vi "Surface_modularity.vi"(2 "Data in":string[][](array[string]), 3 "Channel names":string[](array[string])) -> (0 "Data out":string[][](array[string]))   [LabVIEW 2018]
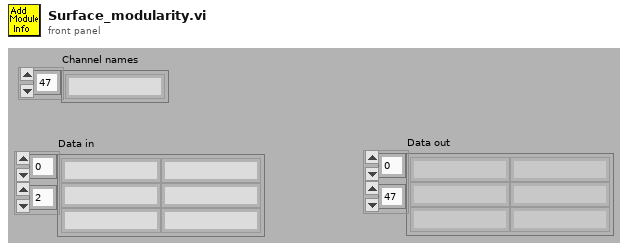
[diagram p1: front panel]
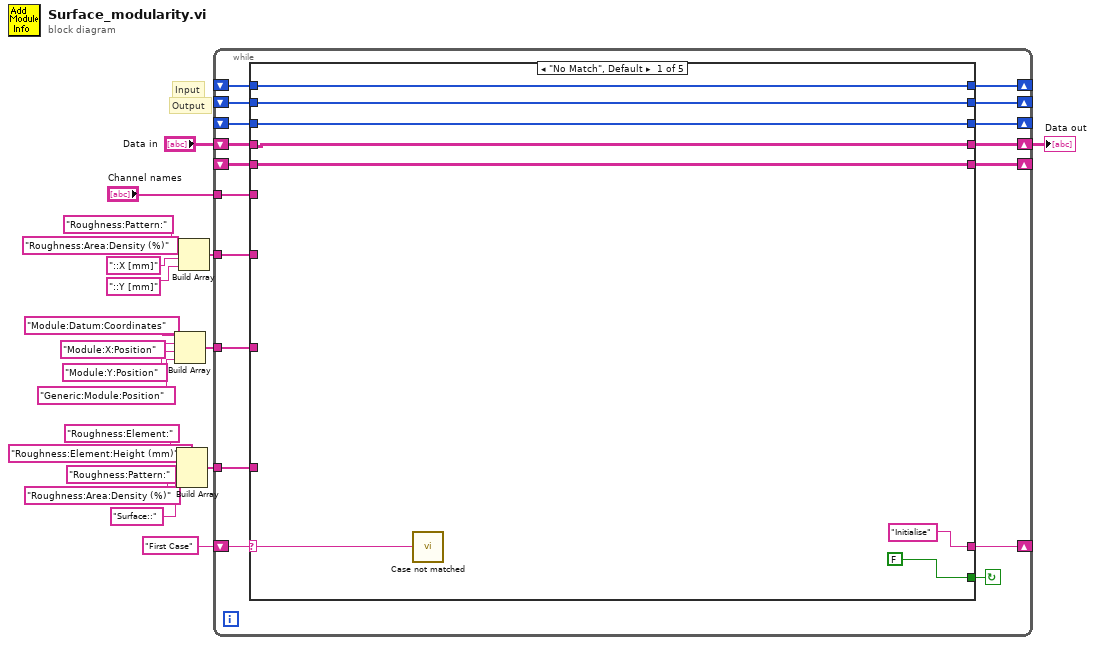
[diagram p0: block diagram]
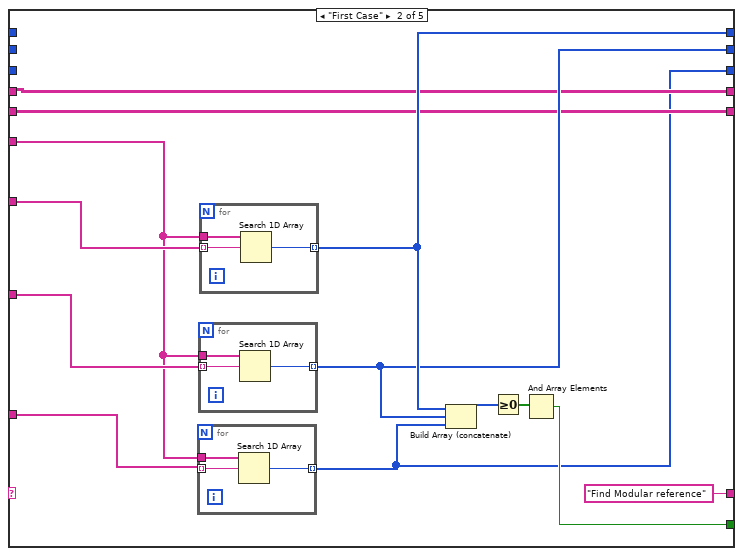
[diagram p2: hidden frame]
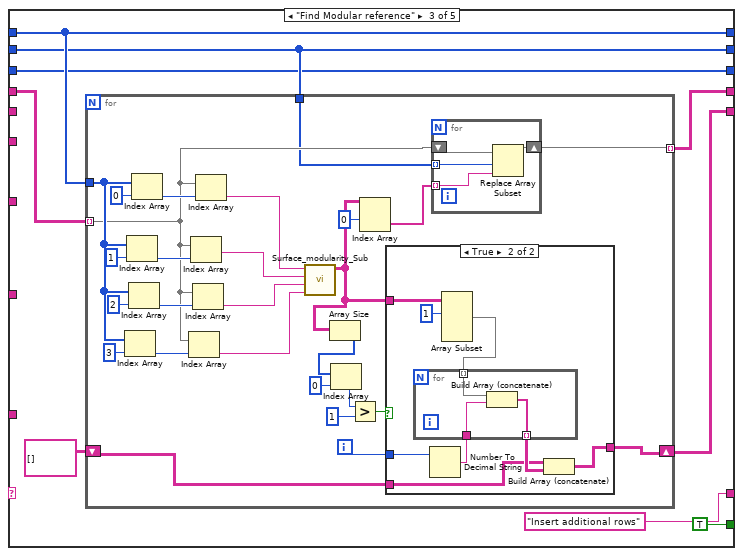
[diagram p3: hidden frame]
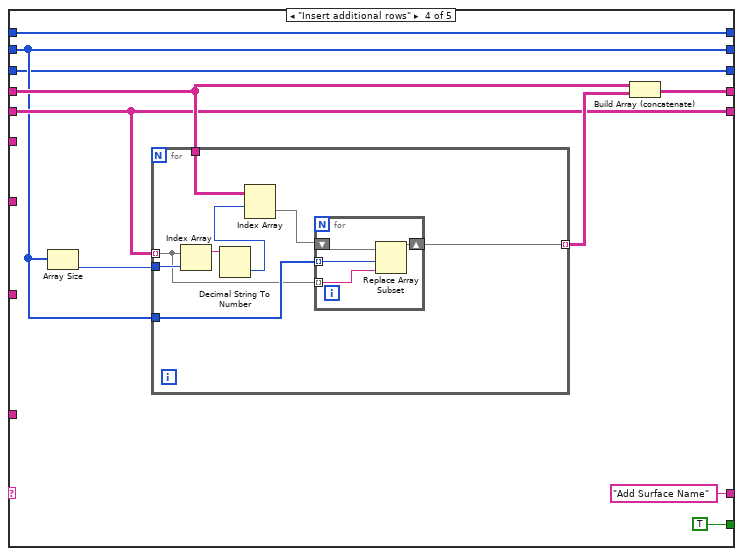
[diagram p5: hidden frame]
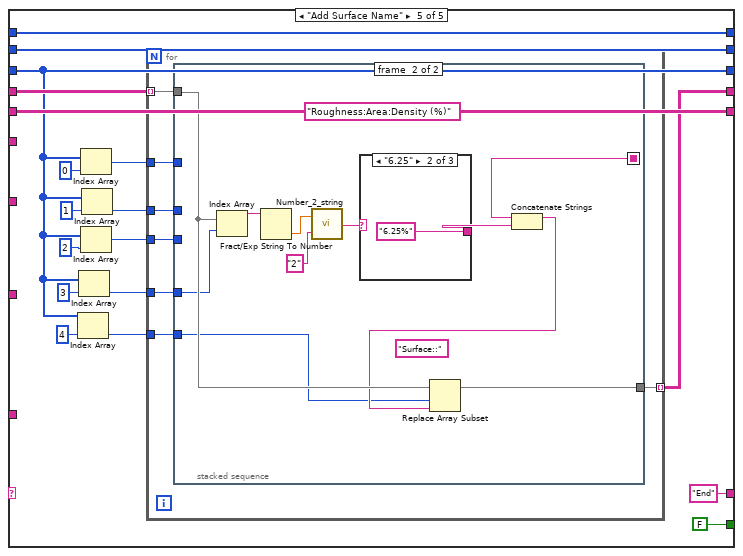
[diagram p6: hidden frame]
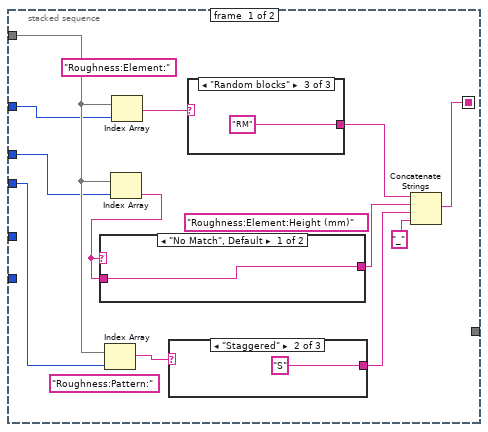
[diagram p7: hidden frame]
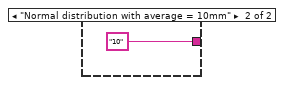
[diagram p8: hidden frame]
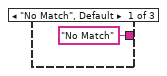
[diagram p9: hidden frame]
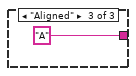
[diagram p10: hidden frame]
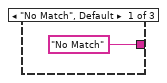
[diagram p11: hidden frame]
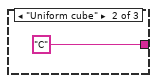
[diagram p12: hidden frame]
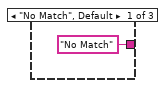
[diagram p13: hidden frame]
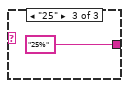
[diagram p14: hidden frame]
diagram:
  # "Output"
  # "Input"
  n1 = Build Array("Module:Datum:Coordinates", "Module:X:Position", "Module:Y:Position", "Generic:Module:Position") -> (w9:string[])
  n2 = Build Array("Roughness:Element:", "Roughness:Element:Height (mm)", "Roughness:Pattern:", "Roughness:Area:Density (%)", "Surface::") -> (w1:string[])
  n3 = Build Array("Roughness:Pattern:", "Roughness:Area:Density (%)", "::X [mm]", "::Y [mm]") -> (w10:string[])
  n4 = while {
    shift-left: "First Case" -> [w35]
    shift-right: [w36] -> _
    shift-right: [w32] -> _
    shift-left: _ -> [w29]
    shift-right: [w30] -> _
    shift-left: _ -> [w28]
    tunnel: "Channel names" -> [w34]
    tunnel: w10 -> [w33]
    tunnel: w9 -> [w31]
    shift-right: [w26] -> w7
    shift-left: "Data in" -> [w27]
    shift-right: [w25] -> _
    shift-left: _ -> [w24]
    tunnel: w1 -> [w23]
    shift-right: [w22] -> _
    shift-left: _ -> [w21]
    stop <- w37 continue-if-true
    n5 = case shown="\"No Match\", Default" w35 {
      selector: w35 -> [w38 _ _ _ _]
      tunnel: [FALSE w50 TRUE TRUE FALSE] -> w37
      tunnel: ["Initialise" "Find Modular reference" "Insert additional rows" "Add Surface Name" "End"] -> w36
      tunnel: w34 -> [_ w48 _ _ _]
      tunnel: w33 -> [_ w57 _ _ _]
      tunnel: [w43 w55 w75 w129 w159] -> w32
      tunnel: w31 -> [_ w56 _ _ _]
      tunnel: [w42 w54 w74 w123 w155] -> w30
      tunnel: w29 -> [w43 _ w75 w129 w159]
      tunnel: w28 -> [w42 _ w74 w123 w155]
      tunnel: w27 -> [w41 w51 w76 w126 w154]
      tunnel: [w41 w51 w71 w125 w153] -> w26
      tunnel: [w40 w49 w69 w124 w156] -> w25
      tunnel: w24 -> [w40 w49 _ w124 w156]
      tunnel: w23 -> [_ w47 _ _ _]
      tunnel: [w39 w46 w68 w120 w142] -> w22
      tunnel: w21 -> [w39 _ w68 w120 w142]
      frame "No Match", Default {
        n6 = call "Case not matched.vi"("Case Name not Matched"=w38) -> ()
      }
      frame "First Case" {
        n7 = for {
          tunnel: w48 -> [w61]
          tunnel: w47 -> [w60] mode=indexing
          tunnel: [w59] -> w46 mode=indexing
          n8 = Search 1D Array(1D array=w61, element=w60) -> (index of element=w59:i32)  [unwired: 1 out]
        }
        n9 = for {
          tunnel: w48 -> [w64]
          tunnel: w56 -> [w63] mode=indexing
          tunnel: [w62] -> w54 mode=indexing
          n10 = Search 1D Array(1D array=w64, element=w63) -> (index of element=w62:i32)  [unwired: 1 out]
        }
        n11 = for {
          tunnel: w48 -> [w67]
          tunnel: w57 -> [w66] mode=indexing
          tunnel: [w65] -> w55 mode=indexing
          n12 = Search 1D Array(1D array=w67, element=w66) -> (index of element=w65:i32)  [unwired: 1 out]
        }
        n13 = Build Array (concatenate)(w55, w54, w46) -> (w53:i32[])
        n14 = Greater Or Equal To 0?(x=w53) -> (x >= 0?=w52:bool[])
        n15 = And Array Elements(Boolean array=w52) -> (logical AND=w50:bool)
      }
      frame "Find Modular reference" {
        n16 = for {
          tunnel: w75 -> [w95]
          tunnel: w76 -> [w94] mode=indexing
          tunnel: w74 -> [w91]
          tunnel: [w88] -> w71 mode=indexing
          shift-right: [w79] -> w69
          shift-left: string[][] [] -> [w80]
          i -> [w81]
          n17 = Index Array(array=w95, index=3) -> (element=w97:i32)
          n18 = Index Array(array=w95, index=1) -> (element=w101:i32)
          n19 = Index Array(array=w95, index=2) -> (element=w98:i32)
          n20 = Index Array(array=w95, index=0) -> (element=w102:i32)
          n21 = Index Array(array=w94, index=w97) -> (element=w77:string)
          n22 = Index Array(array=w94, index=w101) -> (element=w92:string)
          n23 = Index Array(array=w94, index=w98) -> (element=w78:string)
          n24 = Index Array(array=w94, index=w102) -> (element=w93:string)
          n25 = call "Surface_modularity_Sub.vi"("Y Position"=w77, "X Position"=w78, "Roughness Density"=w92, "Roughness Pattern"=w93) -> ("Output values"=w82:string[][])  [unwired: 1 in, 3 out]
          n26 = Array Size(array=w82) -> (size(s)=w87:i32[])
          n27 = Index Array(array=w87, index=0) -> (element=w85:i32)
          n28 = Greater?(x=w85, y=1) -> (0:w83:bool)
          n29 = Index Array(array=w82, index (row)=0) -> (element=w89:string[])  [unwired: 1 in]
          n30 = case shown="True" w83 {
            tunnel: w82 -> [_ w112]
            tunnel: w81 -> [_ w109]
            tunnel: w80 -> [w104 w105]
            tunnel: [w104 w106] -> w79
            frame False {
            }
            frame True {
              n31 = Number To Decimal String(number=w109) -> (decimal integer string=w108:string)  [unwired: 1 out]
              n32 = Array Subset(array=w112, index (row)=1 ("index")) -> (w110:string[][])  [unwired: 3 in]
              n33 = for {
                tunnel: w110 -> [w115] mode=indexing
                tunnel: w108 -> [w114]
                tunnel: [w113] -> w107 mode=indexing
                n34 = Build Array (concatenate)(w115, w114) -> (w113:string[])
              }
              n35 = Build Array (concatenate)(w105, w107) -> (w106:string[][])
            }
          }
          n36 = for {
            shift-right: [w118] -> w88
            shift-left: w94 -> [w119]
            tunnel: w91 -> [w117] mode=indexing
            tunnel: w89 -> [w116] mode=indexing
            n37 = Replace Array Subset(array=w119, new element=w116, index=w117) -> (w118:string[])
          }
        }
      }
      frame "Insert additional rows" {
        n38 = Array Size(array=w123) -> (size(s)=w128:i32)
        n39 = for {
          tunnel: w128 -> [w137]
          tunnel: w124 -> [w131] mode=indexing
          tunnel: w126 -> [w130]
          tunnel: [w133] -> w127 mode=indexing
          tunnel: w123 -> [w132]
          n40 = Index Array(array=w131, index=w137) -> (element=w136:string)
          n41 = Decimal String To Number(string=w136) -> (number=w135:i32)  [unwired: 3 out]
          n42 = Index Array(array=w130, index (row)=w135) -> (element=w134:string[])  [unwired: 1 in]
          n43 = for {
            shift-right: [w140] -> w133
            shift-left: w134 -> [w141]
            tunnel: w132 -> [w139] mode=indexing
            tunnel: w131 -> [w138] mode=indexing
            n44 = Replace Array Subset(array=w141, new element=w138, index=w139) -> (w140:string[])
          }
        }
        n45 = Build Array (concatenate)(w126, w127) -> (w125:string[][])
      }
      frame "Add Surface Name" {
        n46 = Index Array(array=w142, index=4) -> (element=w143:i32)
        n47 = Index Array(array=w142, index=3) -> (element=w144:i32)
        n48 = Index Array(array=w142, index=0) -> (element=w147:i32)
        n49 = Index Array(array=w142, index=2) -> (element=w145:i32)
        n50 = Index Array(array=w142, index=1) -> (element=w146:i32)
        n51 = for {
          tunnel: w154 -> [w166] mode=indexing
          tunnel: [w165] -> w153 mode=indexing
          tunnel: w147 -> [w164]
          tunnel: w146 -> [w163]
          tunnel: w145 -> [w162]
          tunnel: w144 -> [w161]
          tunnel: w143 -> [w160]
          n52 = stacked-sequence {
            seq-local: [w172 _] -> [_ w197]
            tunnel: w166 -> [w175 w195]
            tunnel: [_ w193] -> w165
            tunnel: w164 -> [w171 _]
            tunnel: w163 -> [w170 _]
            tunnel: w162 -> [w169 _]
            tunnel: w161 -> [_ w192]
            tunnel: w160 -> [_ w191]
            frame #0 {
              (unwired) "Roughness:Element:Height (mm)"
              (unwired) "Roughness:Pattern:"
              (unwired) "Roughness:Element:"
              n53 = Index Array(array=w175, index=w169) -> (element=w176:string)
              n54 = Index Array(array=w175, index=w170) -> (element=w167:string)
              n55 = case shown="\"No Match\", Default" w167 {
                tunnel: [w179 "10"] -> w168
                tunnel: w167 -> [w179 _]
                frame "No Match", Default {
                }
                frame "Normal distribution with average = 10mm" {
                }
              }
              n56 = Index Array(array=w175, index=w171) -> (element=w174:string)
              n57 = case shown="\"Staggered\"" w176 {
                tunnel: ["No Match" "S" "A"] -> w177
                frame "No Match", Default {
                }
                frame "Staggered" {
                }
                frame "Aligned" {
                }
              }
              n58 = case shown="\"Random blocks\"" w174 {
                tunnel: ["No Match" "C" "RM"] -> w178
                frame "No Match", Default {
                }
                frame "Uniform cube" {
                }
                frame "Random blocks" {
                }
              }
              n59 = Concatenate Strings(w178, w168, w177, "_") -> (w172:string)
            }
            frame #1 {
              (unwired) "Surface::"
              (unwired) "Roughness:Area:Density (%)"
              n60 = Index Array(array=w195, index=w192) -> (element=w190:string)
              n61 = Fract/Exp String To Number(string=w190) -> (number=w189:dbl)  [unwired: 4 out]
              n62 = call "Number_2_string.vi"("precision"="2", "number"=w189) -> ("String"=w188:string)
              n63 = case shown="\"6.25\"" w188 {
                tunnel: ["No Match" "6.25%" "25%"] -> w196
                frame "No Match", Default {
                }
                frame "6.25" {
                }
                frame "25" {
                }
              }
              n64 = Concatenate Strings(w197, w196) -> (w194:string)
              n65 = Replace Array Subset(array=w195, new element=w194, index=w191) -> (w193:string[])
            }
          }
        }
      }
    }
  }
  "Data out" <- w7
